vi "Find Top Level Panel.vi"(10 "VI (Caller)":string) -> (1 "Found?":bool, 2 "Top Level Panel":string)   [LabVIEW 2020, in "Panel.lvlib" / "Panel.lvclass"]
doc: "Tries to find the top level panel for the specified VI.\n\n<B>VI (Caller):</B> Name of the VI from which to start searching for top-level\n\n<B>Top Level Panel:</B> The name of the top-level panel associated with the input vi name.\n<B>Found:</B> Indicates if the top-level VI was found.\n----\nPlease see the following web address for additional documentation and tutorial information:\nhttp://www.mooregoodideas.com/mgi-panel-manager/\n\nAuthor: Derek Trepanier\n\nCopyright (c) 2018, Moore Good Ideas, Inc.\n\nAll rights reserved.\n\nRedistribution and use in source and binary forms, with or without modification, are permitted provided that the following conditions are met:\n\n * Redistributions of source code must retain the above copyright notice, this list of conditions and the following disclaimer.\n * Redistributions in binary form must reproduce the above copyright notice, this list of conditions and the following disclaimer in the documentation and/or other materials provided with the distribution.\n * Neither the name of Moore Good Ideas, Inc. nor the names of its contributors may be used to endorse or promote products derived from this software without specific prior written permission.\n\nTHIS SOFTWARE IS PROVIDED BY THE COPYRIGHT HOLDERS AND CONTRIBUTORS \"AS IS\" AND ANY EXPRESS OR IMPLIED WARRANTIES, INCLUDING, BUT NOT LIMITED TO, THE IMPLIED WARRANTIES OF MERCHANTABILITY AND FITNESS FOR A PARTICULAR PURPOSE ARE DISCLAIMED. IN NO EVENT SHALL THE COPYRIGHT OWNER OR CONTRIBUTORS BE LIABLE FOR ANY DIRECT, INDIRECT, INCIDENTAL, SPECIAL, EXEMPLARY, OR CONSEQUENTIAL DAMAGES (INCLUDING, BUT NOT LIMITED TO, PROCUREMENT OF SUBSTITUTE GOODS OR SERVICES; LOSS OF USE, DATA, OR PROFITS; OR BUSINESS INTERRUPTION) HOWEVER CAUSED AND ON ANY THEORY OF LIABILITY, WHETHER IN CONTRACT, STRICT LIABILITY, OR TORT (INCLUDING NEGLIGENCE OR OTHERWISE) ARISING IN ANY WAY OUT OF THE USE OF THIS SOFTWARE, EVEN IF ADVISED OF THE POSSIBILITY OF SUCH DAMAGE."
uses:
  <vilib>/MGI/Panel Manager/Panel/Panel/Panel.lvclass
  <vilib>/MGI/Panel Manager/Panel/Panel Registry/Panel Registry.lvclass
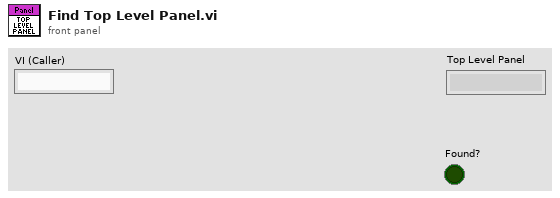
[diagram p1: front panel]
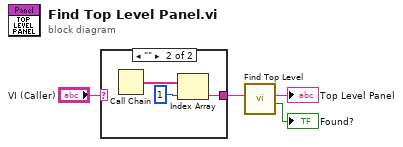
[diagram p0: block diagram]
diagram:
  n1 = case shown="\"\"" "VI (Caller)" {
    selector: "VI (Caller)" -> [w5 _]
    tunnel: [w5 w7] -> w3
    frame Default {
    }
    frame "" {
      n2 = Call Chain() -> (call chain=w8:string[])
      n3 = Index Array(array=w8, index=1) -> (element=w7:string)
    }
  }
  n4 = call <vilib>:"Find Top Level.vi"("VI"=w3) -> ("Found?"=→"Found?":bool, "Top Level Panel"=→"Top Level Panel":string)  [unwired: 8 in, 1 out]
